vi "Write to different sheet LV2012.vi"   [LabVIEW 2016]
doc: "This example creates a new workbook, inserts a numerical table and calls the Excel Set Cell Format VI to customize the cell number format. \n\nThe VI formats the used section of the spreadsheet so that values lower than 0.5 display in blue, and the values greater than 0.5 display in red.\n\nRefer to the Excel documentation for more information about number format."
uses:
  <vilib>/Utility/NIReport.llb/Append Numeric Table to Report (wrap).vi
  <vilib>/Utility/NIReport.llb/NI_report.lvclass
  <vilib>/Utility/NIReport.llb/Excel/NI_Excel.lvclass
panel:
  # "This example creates a new workbook, inserts a numerical table and calls the Excel Set Cell Format VI to customize the cell number format. \n\nThe VI formats the used section of the spreadsheet so that values lower than 0.5 display in red, and the values greater than 0.5 display in blue.\n\nRefer to the Excel documentation for more information about number format."
types:
  T1 = enum16{"Standard Report", "HTML", "Word", "Excel"}
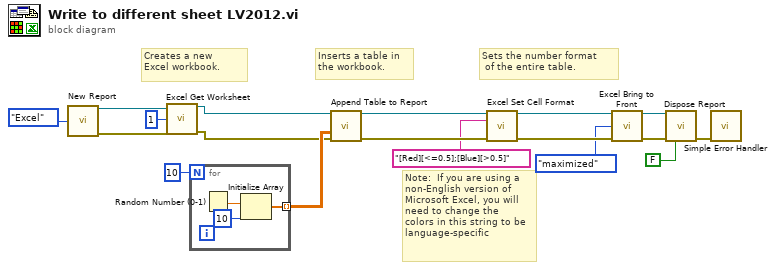
[diagram p0: block diagram]
diagram:
  # "Sets the number format\n of the entire table."
  # "Inserts a table in \nthe workbook."
  # "Creates a new \nExcel workbook."
  # "Note:  If you are using a\nnon-English version of\nMicrosoft Excel, you will\nneed to change the\ncolors in this string to be\nlanguage-specific"
  n1 = call <vilib>:"New Report.vi"("report type"=T1."Excel") -> ("report out"=w3:refnum<class "NI_report.lvclass">, "error out"=w2:errorcluster)  [unwired: 5 in, 8 out]
  n2 = call <vilib>:"Excel Get Worksheet.vi"("report in"=w3, "worksheet index (0)"=1, "error in (no error)"=w2) -> ("report out"=w5:refnum<class "NI_report.lvclass">, "error out"=w4:errorcluster)  [unwired: 11 out]
  n3 = for {
    N: 10 -> [_]
    tunnel: [w19] -> w18 mode=indexing
    n4 = Random Number (0-1)() -> (number: 0 to 1=w21:dbl)
    n5 = Initialize Array(w21, 10 ("dimension size")) -> (w19:dbl[])
  }
  n6 = call-poly <vilib>:"Append Table to Report.vi"("report in"=w5, "numerical data"=w18, "error in (no error)"=w4) -> ("report out"=w15:refnum<class "NI_report.lvclass">, "error out"=w16:errorcluster)  [unwired: 7 in, 4 out]
  n7 = call <vilib>:"Excel Set Cell Format.vi"("report in"=w15, "number format"="[Red][<=0.5];[Blue][>0.5]", "error in (no error)"=w16) -> ("report out"=w11:refnum<class "NI_report.lvclass">, "error out"=w12:errorcluster)  [unwired: 2 in, 9 out]
  n8 = call <vilib>:"Excel Bring to Front.vi"("report in"=w11, "window state (maximized)"=enum16{"maximized", "minimized", "normal"}."maximized", "error in (no error)"=w12) -> ("report out"=w7:refnum<class "NI_report.lvclass">, "error out"=w9:errorcluster)  [unwired: 11 out]
  n9 = call-dynamic "Dispose Report.vi"("report in"=w7, "error in (no error)"=w9, "close report? (T)"=FALSE ("Close Report? (T)")) -> ("error out"=w8:errorcluster)  [unwired: 2 in, 10 out]
  n10 = call <vilib>:"Simple Error Handler.vi"("error in (no error)"=w8) -> ()  [unwired: 1 in, 8 out]
